vi "Execute Turn.vi"(7 "Player Color":T1, 8 "error in":errorcluster, 9 "Possible Moves":bool[][](array[boolean]), 10 "Board":T3[][](array[typedef]), 11 "Player in":refnum<class "Player.lvclass">) -> (0 "error out":errorcluster, 2 "Choice Coordinates":T2, 3 "Player out":refnum<class "Player.lvclass">)   [LabVIEW 2020, in "Reversi.lvlib" / "Player.lvclass"]
uses:
  Player.lvclass
  Space Coordinates.ctl
  Reversi.lvclass
  <vilib>/numeric/Random Number (Range) I64.vi
  Space Ring.ctl
  Turn Enum.ctl
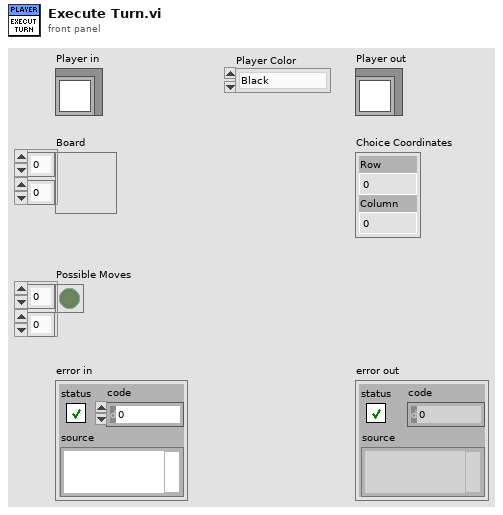
[diagram p1: front panel]
types:
  T1 = typedef "Reversi.lvlib/Reversi.lvclass/Turn Enum.ctl" = enum16{"Black", "White"}
  T2 = typedef "Reversi.lvlib/Reversi.lvclass/Space Coordinates.ctl" = cluster{"Row":i32, "Column":i32}
  T3 = typedef "Reversi.lvlib/Reversi.lvclass/Space Ring.ctl" = u16
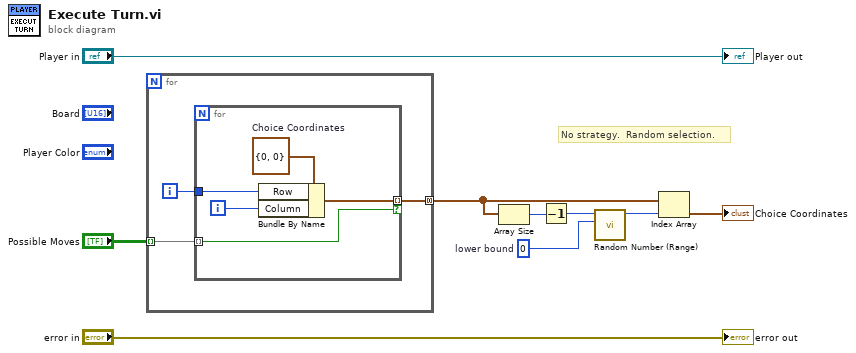
[diagram p0: block diagram]
diagram:
  w2 = i64 0  # lower bound
  # "No strategy.  Random selection."
  n1 = for {
    tunnel: "Possible Moves" -> [w12] mode=indexing
    tunnel: [w10] -> w5 mode=concatenating
    i -> [w11]
    n2 = for {
      tunnel: w12 -> [w13] mode=indexing
      tunnel: w11 -> [w15]
      tunnel: [w14] -> w10 mode=indexing if=w13
      i -> [w16]
      w17 = T2 {"Row"=0, "Column"=0}  # Choice Coordinates
      n3 = Bundle By Name(cluster=w17, "Row"=w15, "Column"=w16) -> (w14:T2)
    }
  }
  n4 = Array Size(array=w5) -> (size(s)=w6:i32)
  n5 = Decrement(x=w6) -> (x-1=w3:i32)
  n6 = call-poly <vilib>:"Random Number (Range).vi"("lower bound (-100)"=w2, "upper bound (100)"=w3) -> ("number"=w1:i64)  [unwired: 9 in]
  n7 = Index Array(array=w5, index=w1) -> (element=→"Choice Coordinates":T2)
  "error out" <- "error in"
  "Player out" <- "Player in"
